vi "EMC_Reset.vi"(8 "error in (no error)":errorcluster, 10 "Position":dbl, 11 "axis":refnum<k21>) -> (0 "error out":errorcluster)   [LabVIEW 2014]
uses:
  EMC_Typedef_Motor_Parameters.ctl
  <resource>/objmgr/nimcca.rc
panel:
  in  "table":refnum<k21>
  in  "coordinate":refnum<k21>
  in  "Motion Parameters":T1={"position"=1000.0, "velocity"=1000.0, "acceleration"=10000.0, "deceleration"=10000.0, "accel. jerk"=10000.0, "decel. jerk"=10000.0}
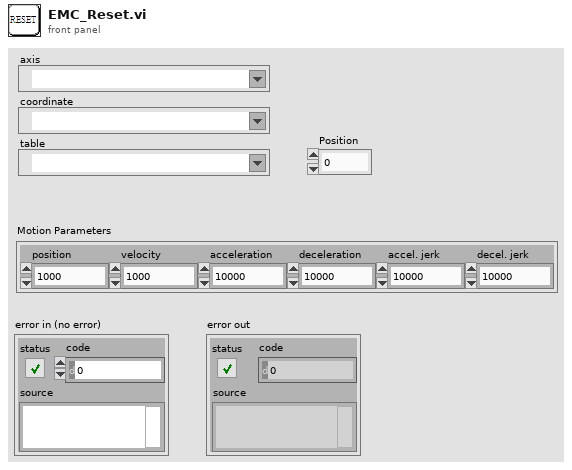
[diagram p1: front panel]
types:
  T1 = typedef "EMC_Typedef_Motor_Parameters.ctl" = cluster{"position":dbl, "velocity":dbl, "acceleration":dbl, "deceleration":dbl, "accel. jerk":dbl, "decel. jerk":dbl}
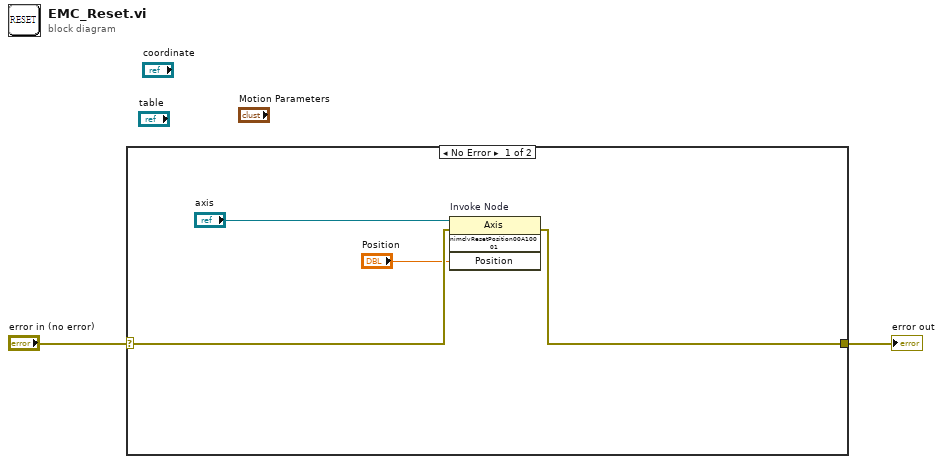
[diagram p0: block diagram]
diagram:
  n1 = case shown="No Error" "error in (no error)" {
    selector: "error in (no error)" -> [w5 w7]
    tunnel: [w4 w7] -> w2
    frame No Error {
      n2 = invoke on="Invoke Node" class="Axis" method="nimclvResetPosition00A10001"(reference="axis", error in=w5, "Position"="Position") -> (error out=w4:errorcluster)  [unwired: 1 in, 3 out]
    }
    frame Error {
    }
  }
  "error out" <- w2
